vi "multiply_1000.vi"(10 "Numeric":dbl) -> (2 "Numeric 2":dbl)   [LabVIEW 2025]
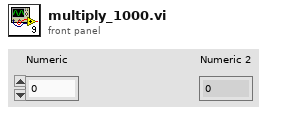
[diagram p1: front panel]
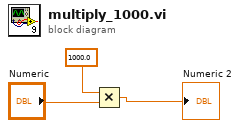
[diagram p0: block diagram]
diagram:
  n1 = Multiply(x=1000.0, y="Numeric") -> (x*y=→"Numeric 2":dbl)
